vi "Async.Engine.Close.vi"(8 "error in":errorcluster, 11 "Async in":refnum<class "VS Inline Async API (Express).lvclass">) -> (0 "error out":errorcluster, 3 "Async out":refnum<class "VS Inline Async API (Express).lvclass">)   [LabVIEW 2026, in "VS Inline Async API (Express).lvlib" / "VS Inline Async API (Express).lvclass"]
uses:
  VS Inline Async API (Express).lvclass
  VS Inline Async API (Express).lvclass/VS Inline Async API (Express).ctl
  _Data Access Engine (Express)/Data Access Engine (Express)/Data Access Engine (Express).lvclass
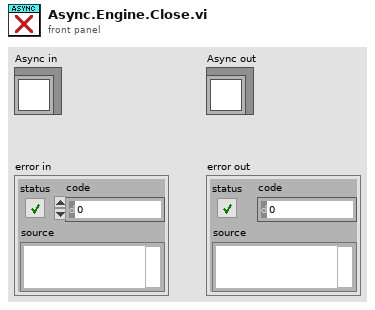
[diagram p1: front panel]
types:
  T1 = typedef "VS Inline Async API (Express).lvlib/VS Inline Async API (Express).lvclass/Error Handling Settings.ctl" = cluster{"Write to SystemLog (F)":bool}
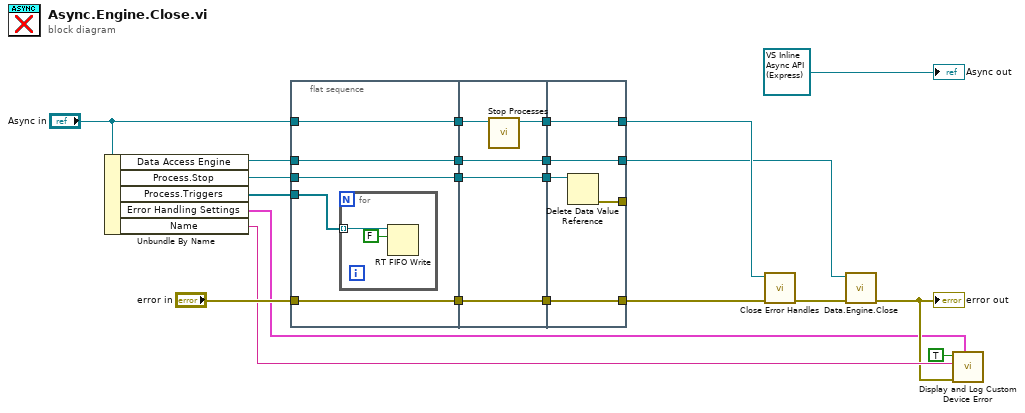
[diagram p0: block diagram]
diagram:
  n1 = Unbundle By Name("Async in") -> ("Data Access Engine"=w9:refnum<class "Data Access Engine (Express).lvclass">, "Process.Stop"=w16:refnum<data-value>, "Process.Triggers"=w8:refnum<k33>[], "Error Handling Settings"=w3:T1, "Name"=w18:string)
  n2 = flat-sequence {
    tunnel: [w27] -> w22
    tunnel: "error in" -> [w27]
    tunnel: [w26] -> w17
    tunnel: "Async in" -> [w26]
    tunnel: w16 -> [w25]
    tunnel: [w25] -> w15
    tunnel: [w24] -> w10
    tunnel: w9 -> [w24]
    tunnel: w8 -> [w23]
    tunnel: [w34] -> w7
    tunnel: w22 -> [w34]
    tunnel: w17 -> [w33]
    tunnel: [w32] -> w6
    tunnel: w15 -> [w32]
    tunnel: [w31] -> w5
    tunnel: [w30] -> w4
    tunnel: w10 -> [w30]
    tunnel: [w39] -> w20
    tunnel: w7 -> [w39]
    tunnel: w6 -> [w38]
    tunnel: [w37] -> w14
    tunnel: w5 -> [w37]
    tunnel: [w36] -> _
    tunnel: [w35] -> w11
    tunnel: w4 -> [w35]
    frame #0 {
      n3 = for {
        tunnel: w23 -> [w29] mode=indexing
        n4 = RT FIFO Write(0:w29, 1:FALSE ("element")) -> ()  [unwired: 3 in, 4 out]
      }
    }
    frame #1 {
      n5 = call "Stop Processes.vi"("Async in"=w33) -> ("Async out"=w31:refnum<class "VS Inline Async API (Express).lvclass">)  [unwired: 10 in]
    }
    frame #2 {
      n6 = Delete Data Value Reference(data value reference=w38) -> (error out=w36:errorcluster)  [unwired: 1 in, 1 out]
    }
  }
  n7 = call "Close Error Handles.vi"("error in"=w20, "Async in"=w14) -> ("error out"=w13:errorcluster)  [unwired: 8 in, 1 out]
  n8 = call "Data.Engine.Close.vi"("error in"=w13, "Data Access API in"=w11) -> ("error out"=w12:errorcluster)  [unwired: 8 in, 1 out]
  "error out" <- w12
  n9 = call "Display and Log Custom Device Error.vi"("Error Log Settings"=w3, "error out"=w12, "Your code's public name"=w18, "Custom Device? (T)"=TRUE) -> ()  [unwired: 8 in]
  "Async out" <- refnum<class "VS Inline Async API (Express).lvclass"> refnum ("Async in")
